vi "Initiate Sample Transfer.vi"(6 "Fail State (Idle)":T1, 7 "Transfer mBar":dbl, 8 "error in (no error)":errorcluster, 9 "Target Container":T2, 10 "Source Container":T2, 11 "cRIO-CO2 in":refnum<class "cRIO-CO2.lvclass">) -> (0 "error out":errorcluster, 1 "Success?":bool, 3 "cRIO-CO2 out":refnum<class "cRIO-CO2.lvclass">)   [LabVIEW 2015, in "cRIO-Carbondioxide.lvlib" / "cRIO-CO2.lvlib" / "cRIO-CO2.lvclass"]
uses:
  cRIO-CO2.lvclass
  Controls/Sample Transfer Container Enumerator.ctl
  Controls/Sample Transfer State Enumerator.ctl
  cRIO-CO2.lvclass/cRIO-CO2.ctl
  <vilib>/ActorFramework/Message Enqueuer/Message Priority.ctl
  Transfer Line/Transfer Line.lvclass
  CO2 Actor Messages/Ping Msg/Ping Msg.lvclass/Ping Msg.ctl
  <vilib>/ActorFramework/Message Enqueuer/Message Enqueuer.lvclass/Message Enqueuer.ctl
  Transfer Line/Transfer Line.lvclass/Transfer Line.ctl
  cRIO-CO2 Messages/Log Message Msg/Log Message Msg.lvclass/Log Message Msg.ctl
  <vilib>/ActorFramework/Message Enqueuer/Enqueue.vi
  State Elapsed Time.vi
  <vilib>/ActorFramework/Message Priority Queue/Priority Enqueue.vi
  subs/Sample/Read Sample From Container.vi
  <vilib>/ActorFramework/Message Enqueuer/Message Enqueuer.lvclass
  CO2 Actor Messages/Ping Msg/Ping Msg.lvclass
  <vilib>/ActorFramework/Actor/Actor.lvclass
  subs/Sample/Sample.lvclass
  cRIO-CO2 Messages/Log Message Msg/Log Message Msg.lvclass
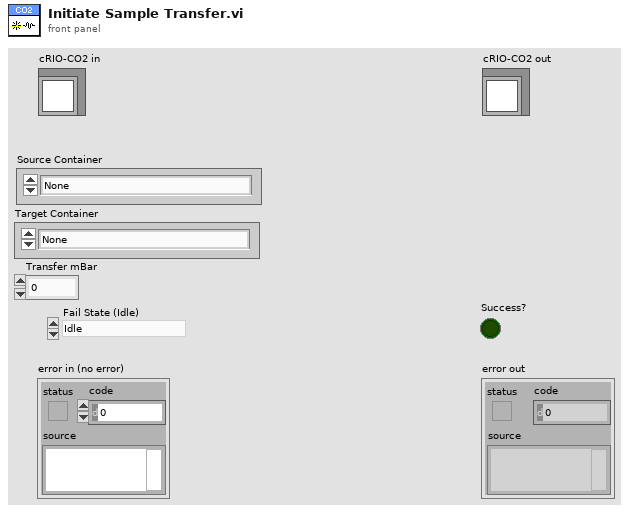
[diagram p1: front panel]
types:
  T1 = typedef "Sample Transfer State Enumerator.ctl" = enum16{"Idle", "Initialize", "Check Containers", "Check Temperatures", "Start Turbo", "Warm Up Containers", "Prepare for purging", "Purge Capillary", "Purge", "Open Containers", "Introduce Sample", "Measure Base Pressure", "Home Syringe", "Start Freezer", "Freeze Target", "Crystalize", "Initiate Stash", "Stash", "Polish", "Stop Freezers", "Push Sample", "Complete", "Abort", "Error", "Undefined"}
  T2 = typedef "Sample Transfer Container Enumerator.ctl" = enum16{"None", "Sample 1", "Sample 2", "Sample 3", "Sample 4", "Sample 5", "Storage 01", "Storage 02", "Storage 03", "Storage 04", "Storage 05", "Storage 06", "Storage 07", "Storage 08", "Storage 09", "Storage 10", "Storage 11", "Storage 12", "Syringe", "Undefined"}
  T3 = typedef "Actor Framework.lvlib/Message Enqueuer.lvclass/Message Priority.ctl" = enum16{"Low", "Normal", "High"}
  T4 = typedef "Sample Push State Enumerator.ctl" = enum16{"Undefined", "Initialize", "Dilute", "Close Transfer Line", "Start Heaters", "Warm Up Syringe", "Ready to Push", "Push", "Initiate Stash", "Stash", "Complete", "Abort", "Idle", "Error"}
  T5 = typedef "Containers Check Enumerator.ctl" = enum16{"Ok", "Same", "Undefined", "Invalid Target", "Invalid Push State", "Invalid Source Sample"}
  T6 = typedef "Dedicated Enqueuers.ctl" = cluster{"Freezers":cluster{"Syringe":refnum<class "Message Enqueuer.lvclass">, "Tank 1":refnum<class "Message Enqueuer.lvclass">, "Tank 2":refnum<class "Message Enqueuer.lvclass">, "Tank 3":refnum<class "Message Enqueuer.lvclass">, "Tank 4":refnum<class "Message Enqueuer.lvclass">}, "Heaters":cluster{"Syringe":refnum<class "Message Enqueuer.lvclass">, "Piston":refnum<class "Message Enqueuer.lvclass">}, "Blowers":cluster{"Tank 1":refnum<class "Message Enqueuer.lvclass">, "Tank 2":refnum<class "Message Enqueuer.lvclass">, "Tank 3":refnum<class "Message Enqueuer.lvclass">, "Tank 4":refnum<class "Message Enqueuer.lvclass">, "Syringe":refnum<class "Message Enqueuer.lvclass">}, "Sample Line":refnum<class "Message Enqueuer.lvclass">, "Storage Line":refnum<class "Message Enqueuer.lvclass">, "Transfer Line":refnum<class "Message Enqueuer.lvclass">, "Syringe Stepper":refnum<class "Message Enqueuer.lvclass">, "Syringe Line":refnum<class "Message Enqueuer.lvclass">, "Capillary Line":refnum<class "Message Enqueuer.lvclass">, "Preparation Line":refnum<class "Message Enqueuer.lvclass">, "Turbo":refnum<class "Message Enqueuer.lvclass">, "Vacuum":refnum<class "Message Enqueuer.lvclass">, "He Line":refnum<class "Message Enqueuer.lvclass">, "Cylinder":refnum<class "Message Enqueuer.lvclass">}
  T7 = typedef "Sample Container.ctl" = cluster{"Sample In":refnum<k21>, "Sample Name":refnum<k21>, "Ti Cathode":refnum<k21>, "SampleQ":refnum<queue>}
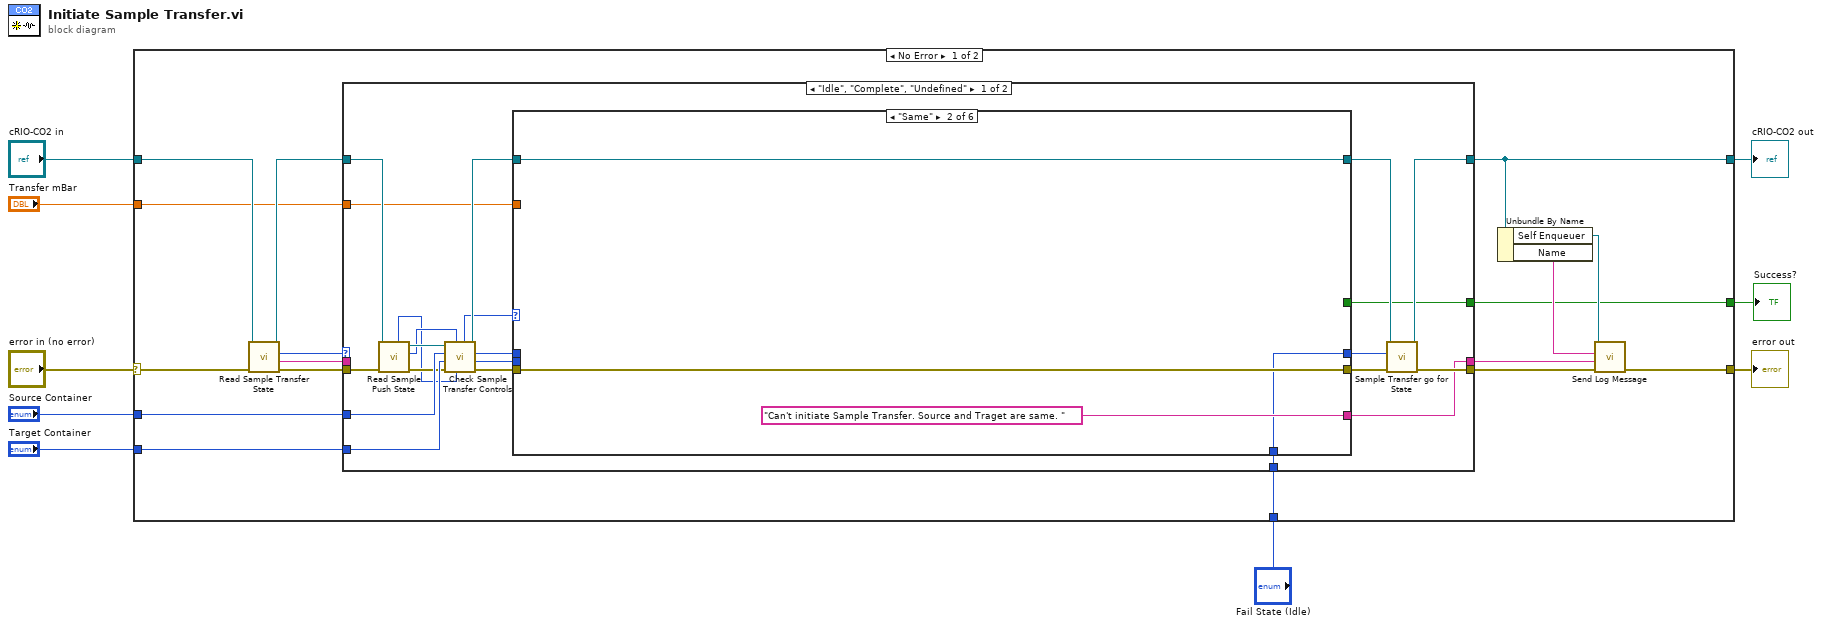
[diagram p0: block diagram]
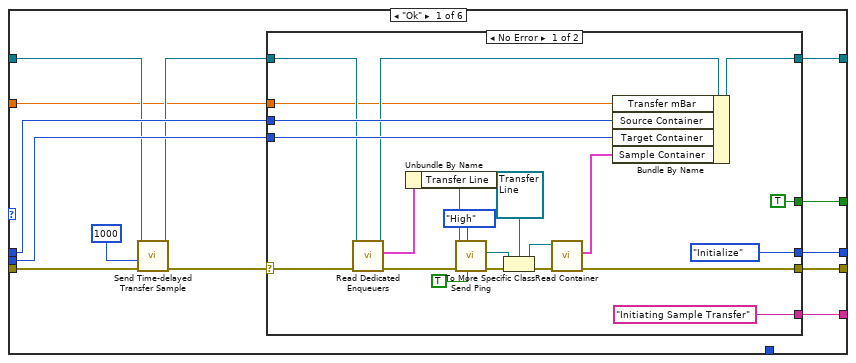
[diagram p2: hidden frame]
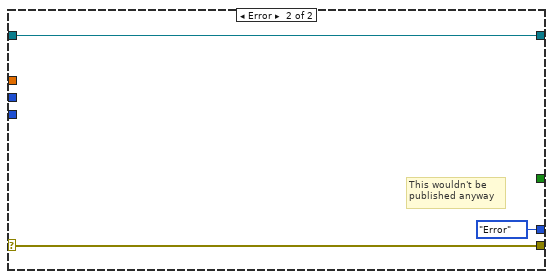
[diagram p3: hidden frame]
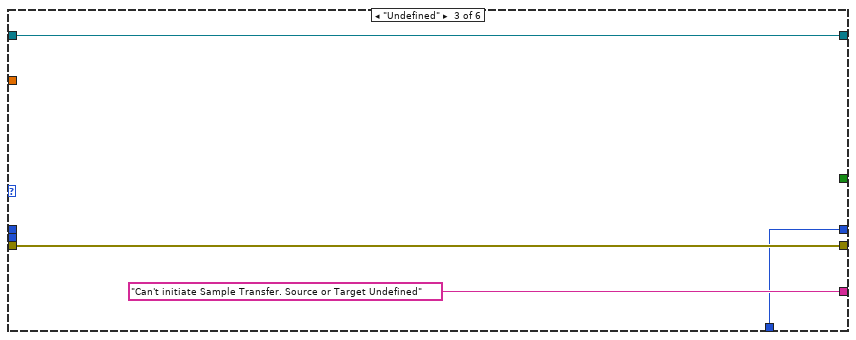
[diagram p4: hidden frame]
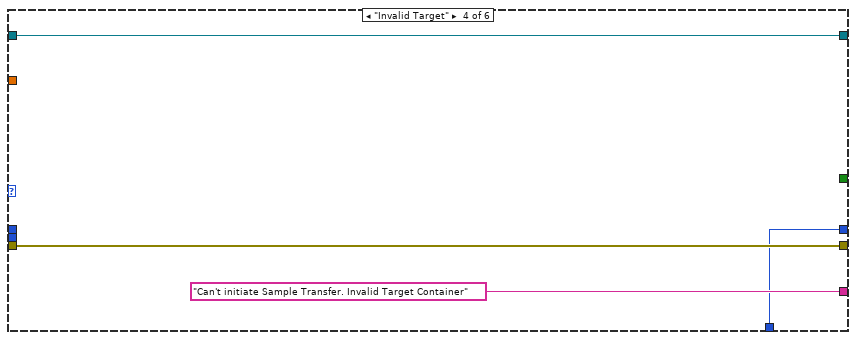
[diagram p5: hidden frame]
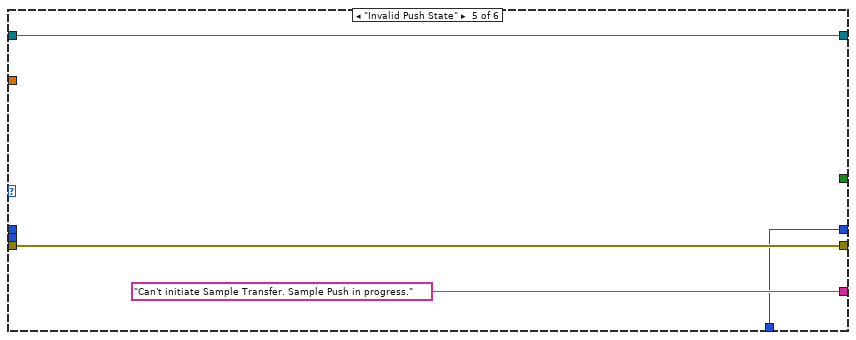
[diagram p6: hidden frame]
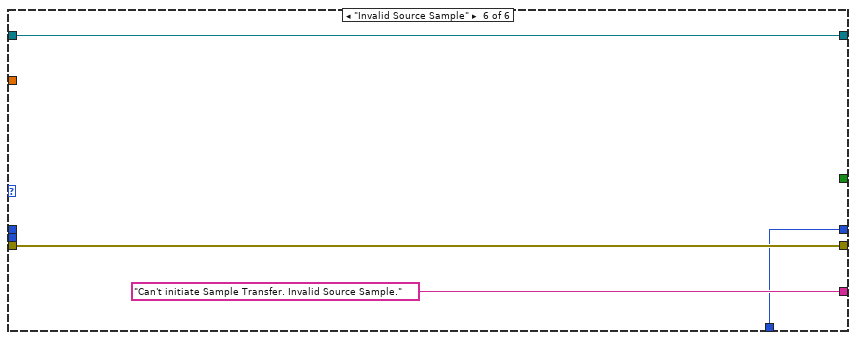
[diagram p7: hidden frame]
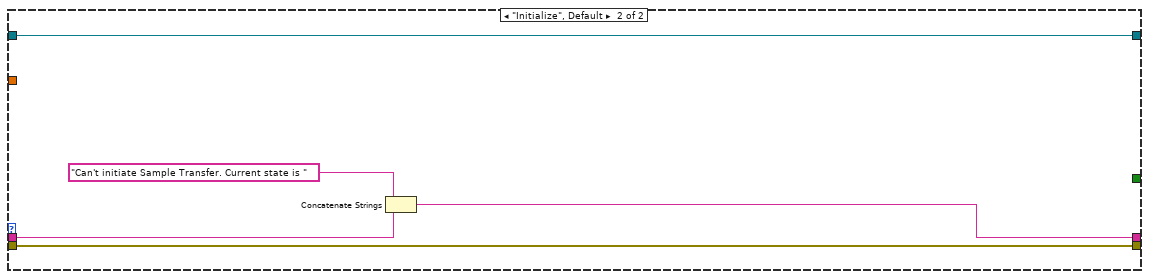
[diagram p8: hidden frame]
diagram:
  n1 = case shown="No Error" "error in (no error)" {
    selector: "error in (no error)" -> [w16 w113]
    tunnel: [w21 w113] -> w8
    tunnel: [w17 w112] -> w6
    tunnel: "cRIO-CO2 in" -> [w15 w112]
    tunnel: "Source Container" -> [w14 _]
    tunnel: "Target Container" -> [w13 _]
    tunnel: "Transfer mBar" -> [w12 _]
    tunnel: "Fail State (Idle)" -> [w11 _]
    tunnel: [w10 _] -> w1
    frame No Error {
      n2 = call "Read Sample Transfer State.vi"("error in (no error)"=w16, "cRIO-CO2 in"=w15) -> ("error out"=w25:errorcluster, 1:"Sample Transfer State"=w23:string, 2:"Sample Transfer State"=w26:T1, "cRIO-CO2 out"=w24:refnum<class "cRIO-CO2.lvclass">)  [unwired: 4 in, 2 out]
      n3 = case shown="\"Idle\", \"Complete\", \"Undefined\"" w26 {
        tunnel: w25 -> [w35 w109]
        tunnel: w24 -> [w33 w108]
        tunnel: [w42 w109] -> w22
        tunnel: w23 -> [_ w107]
        tunnel: [w41 w110] -> w18
        tunnel: [w39 w108] -> w17
        tunnel: w14 -> [w36 _]
        tunnel: w13 -> [w37 _]
        tunnel: w12 -> [w30 _]
        tunnel: w11 -> [w28 _]
        tunnel: [w27 _] -> w10
        frame "Idle", "Complete", "Undefined" {
          n4 = call "Read Sample Push State.vi"("error in (no error)"=w35, "cRIO-CO2 in"=w33) -> ("error out"=w34:errorcluster, "Sample Push State"=w31:T4, "cRIO-CO2 out"=w32:refnum<class "cRIO-CO2.lvclass">, "Source Storage"=w29:T2)  [unwired: 3 in, 3 out]
          n5 = call "Check Sample Transfer Controls.vi"("Push Source Storage"=w29, "Sample Push State"=w31, "error in (no error)"=w34, "Target Container"=w37, "Source Container"=w36, "cRIO-CO2 in"=w32) -> ("error out"=w48:errorcluster, "Target Container"=w45:T2, "Source Container"=w46:T2, "cRIO-CO2 out"=w47:refnum<class "cRIO-CO2.lvclass">, "Containers check"=w44:T5)  [unwired: 1 in]
          n6 = case shown="\"Same\"" w44 {
            tunnel: w48 -> [w52 w89 w93 w97 w101 w105]
            tunnel: [w56 w89 w93 w97 w101 w105] -> w43
            tunnel: w47 -> [w55 w88 w94 w98 w102 w106]
            tunnel: [w60 w88 w94 w98 w102 w106] -> w40
            tunnel: [w61 "Can't initiate Sample Transfer. Source and Traget are same. " "Can't initiate Sample Transfer. Source or Target Undefined" "Can't initiate Sample Transfer. Invalid Target Container" "Can't initiate Sample Transfer. Sample Push in progress." "Can't initiate Sample Transfer. Invalid Source Sample."] -> w41
            tunnel: w46 -> [w59 _ _ _ _ _]
            tunnel: w45 -> [w58 _ _ _ _ _]
            tunnel: [w53 w87 w91 w95 w99 w103] -> w38
            tunnel: w30 -> [w50 _ _ _ _ _]
            tunnel: w28 -> [_ w87 w91 w95 w99 w103]
            tunnel: [w49 _ _ _ _ _] -> w27
            frame "Ok" {
              n7 = call "Send Time-delayed Transfer Sample.vi"("error in (no error)"=w52, "Milliseconds To Wait (1000)"=1000, "cRIO-CO2 in"=w55) -> ("error out"=w57:errorcluster, "cRIO-CO2 out"=w54:refnum<class "cRIO-CO2.lvclass">)  [unwired: 7 in]
              n8 = case shown="No Error" w57 {
                selector: w57 -> [w65 w85]
                tunnel: ["Initiating Sample Transfer" _] -> w61
                tunnel: [w82 w86] -> w60
                tunnel: w59 -> [w81 _]
                tunnel: w58 -> [w80 _]
                tunnel: [w72 w85] -> w56
                tunnel: w54 -> [w66 w86]
                tunnel: [Sample_Transfer_State_Enumerator."Initialize" ("Sample Transfer State") Sample_Transfer_State_Enumerator."Error" ("Sample Transfer State")] -> w53
                tunnel: w50 -> [w63 _]
                tunnel: [TRUE _] -> w49
                frame No Error {
                  n9 = call "Read Dedicated Enqueuers.vi"("error in (no error)"=w65, "cRIO-CO2 in"=w66) -> ("error out"=w77:errorcluster, "Dedicated Enqueuers"=w78:T6, "cRIO-CO2 out"=w79:refnum<class "cRIO-CO2.lvclass">)  [unwired: 6 in, 1 out]
                  n10 = Unbundle By Name(w78) -> ("Transfer Line"=w76:refnum<class "Message Enqueuer.lvclass">)
                  n11 = call "Send Ping.vi"("Return Self (F)"=TRUE, "Message Priority (Normal)"=Message_Priority."High", "error in (no error)"=w77, "Message Enqueuer"=w76) -> ("error out"=w73:errorcluster, "Actor out"=w70:refnum<class "Actor.lvclass">)  [unwired: 4 in, 2 out]
                  n12 = To More Specific Class(target class=refnum<class "Transfer Line.lvclass"> refnum ("Transfer Line in"), reference=w70, error in=w73) -> (specific class reference=w68:refnum<class "Transfer Line.lvclass">, error out=w71:errorcluster)
                  n13 = call "Read Container.vi"("error in (no error)"=w71, "Transfer Line in"=w68) -> ("error out"=w72:errorcluster, "Sample Container"=w67:T7)  [unwired: 5 in, 3 out]
                  n14 = Bundle By Name(cluster=w79, "Transfer mBar"=w63, "Source Container"=w81, "Target Container"=w80, "Sample Container"=w67) -> (w82:refnum<class "cRIO-CO2.lvclass">)
                }
                frame Error {
                  # "This wouldn't be\npublished anyway"
                }
              }
            }
            frame "Same" {
            }
            frame "Undefined" {
            }
            frame "Invalid Target" {
            }
            frame "Invalid Push State" {
            }
            frame "Invalid Source Sample" {
            }
          }
          n15 = call "Sample Transfer go for State.vi"("error in (no error)"=w43, "Sample Transfer State"=w38, "cRIO-CO2 in"=w40) -> ("error out"=w42:errorcluster, "cRIO-CO2 out"=w39:refnum<class "cRIO-CO2.lvclass">)  [unwired: 7 in]
        }
        frame "Initialize", Default {
          n16 = Concatenate Strings("Can't initiate Sample Transfer. Current state is ", w107) -> (w110:string)
        }
      }
      n17 = Unbundle By Name(w17) -> ("Self Enqueuer"=w20:refnum<class "Message Enqueuer.lvclass">, "Name"=w19:string)
      n18 = call "Send Log Message.vi"("error in (no error)"=w22, "String"=w18, "Source Name"=w19, "Message Enqueuer"=w20) -> ("error out"=w21:errorcluster)  [unwired: 6 in, 1 out]
    }
    frame Error {
    }
  }
  "error out" <- w8
  "cRIO-CO2 out" <- w6
  "Success?" <- w1
